vi "TagDB-TestMain2(ouside).vi"() -> ()   [LabVIEW 2017]
uses:
  438369a8-d9b2-41af-8945-45e8f27329f7.vi
  d53a7300-4718-4e6c-94be-b335989d07a0.vi
  src/TagDB/_Support/DataAccess/_NameCacher.vi
  src/TagDB/_Support/Error/_[error50002]Invalid DataType.vi
  src/TagDB/_Support/Error/_[error50000]Invalid DB REF.vi
  src/TagDB/_Support/DataAccess/TagDB Ref to DVR.vi
  src/TagDB/_Support/URL/TRIM-BOTH-SPACE.vi
  src/TagDB/_Support/DataAccess/data-Write.vi
  src/TagDB/_Support/DataAccess/_datatypeChecker.vi
  <vilib>/Utility/Data Type/Get Type Information.vi
  src/TagDB/_Support/Error/_Build Error Cluster.vi
  src/TagDB/TagDB.lvlib
panel:
  in  "name (unnamed)":string="db"
  in  "write tag":string="abc"
  in  "Numeric":i32=123124312
  in  "read tag":string="abc"
  out "Value":variant
  in  "stop":bool
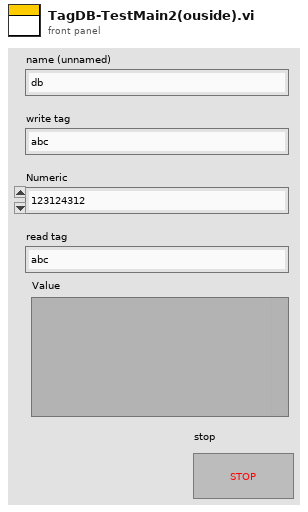
[diagram p1: front panel]
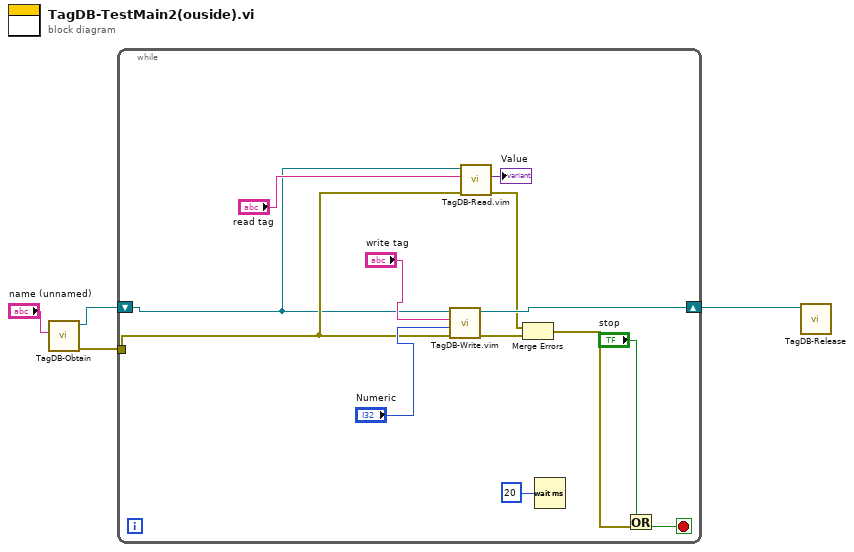
[diagram p0: block diagram]
diagram:
  n1 = call "TagDB-Obtain.vi"("name (unnamed)"="name (unnamed)") -> ("error out"=w4:errorcluster, "TagDB"=w3:refnum<k1>)  [unwired: 4 in, 1 out]
  n2 = while {
    tunnel: w4 -> [w12]
    shift-right: [w15] -> w1
    shift-left: w3 -> [w11]
    stop <- w8 stop-if-true
    n3 = call "TagDB-Write.vim"("error in (no error)"=w12, "Value"="Numeric", "tag"="write tag", "TagDB"=w11) -> ("error out"=w14:errorcluster, "TagDB(dup)"=w15:refnum<k1>)  [unwired: 5 in, 1 out]
    n4 = call "TagDB-Read.vim"("error in (no error)"=w12, "name"="read tag", "TagDB"=w11) -> ("error out"=w5:errorcluster, "Value"=→"Value":variant)  [unwired: 3 in, 4 out]
    n5 = Merge Errors(w5, w14) -> (w6:errorcluster)
    n6 = Wait (ms)(milliseconds to wait=u32 20 ("millisecond timer value")) -> ()  [unwired: 1 out]
    n7 = Or(x="stop", y=w6) -> (x .or. y?=w8:bool)
  }
  n8 = call "TagDB-Release.vi"("TagDB"=w1) -> ()  [unwired: 10 in, 1 out]
